vi "AMB_Monitor.vi"(0 "ObjHandle in":u32, 1 "CAN ID in":u32 format="%.0x", 2 "error in":errorcluster {"code" format="%.0x"}) -> (3 "ObjHandle out":u32, 4 "Data Array out":u8[](array[numeric]) format="%.0x", 5 "Data Length out":u8, 6 "error out":errorcluster {"code" format="%.0x"})   [LabVIEW 2017]
doc: "ALMA M&C Bus Read Monitor\nGets a monitor value on the specified CAN ID\nFirst clears the read queue of any stale messages\ntransmits the monitor requests and waits up to 2ms\nfor a response. Timeout is signalled in error cluster."
panel:
  # "AMB Monitor and Control Bus\nGet Monitor Data"
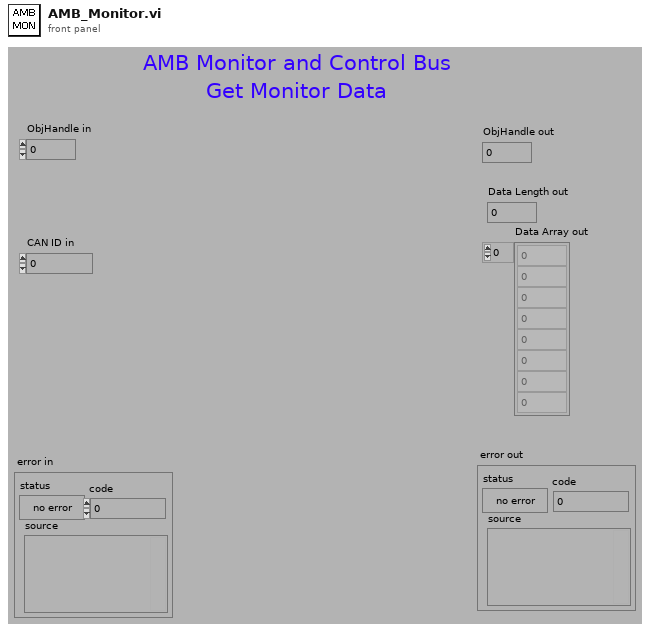
[diagram p1: front panel]
types:
  T1 = typedef "xobjhandle.ctl" = u32
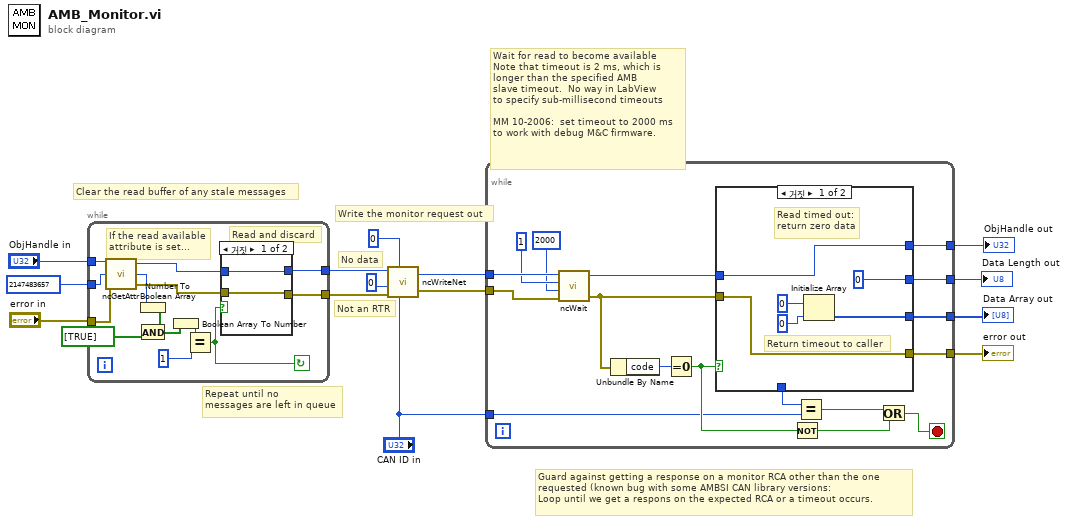
[diagram p0: block diagram]
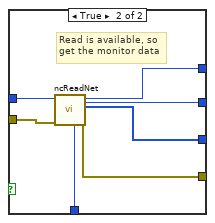
[diagram p2: hidden frame]
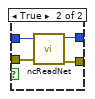
[diagram p3: hidden frame]
diagram:
  # "Guard against getting a response on a monitor RCA other than the one \nrequested (known bug with some AMBSI CAN library versions:\nLoop until we get a respons on the expected RCA or a timeout occurs."
  # "Wait for read to become available\nNote that timeout is 2 ms, which is\nlonger than the specified AMB\nslave timeout.  No way in LabView\nto specify sub-millisecond timeouts\n\nMM 10-2006:  set timeout to 2000 ms\nto work with debug M&C firmware."
  # "Not an RTR"
  # "No data"
  # "Write the monitor request out"
  # "Repeat until no\nmessages are left in queue"
  # "Clear the read buffer of any stale messages"
  n1 = while {
    tunnel: u32 2147483657 -> [w15]
    tunnel: [w22] -> w3
    tunnel: [w23] -> w4
    tunnel: "error in" -> [w27]
    tunnel: "ObjHandle in" -> [w28]
    stop <- w21 continue-if-true
    # "Read and discard"
    # "If the read available\nattribute is set..."
    n2 = call <vilib>:"ncGetAttr.vi"("Error in"=w27, "AttrId"=w15, "ObjHandle in"=w28) -> ("Error out"=w24:errorcluster, "AttrValue"=w20:u32, "ObjHandle out"=w25:T1)
    n3 = Number To Boolean Array(number=w20) -> (Boolean array=w19:bool[])
    n4 = And(x=w19, y=bool[] [TRUE]) -> (x .and. y?=w17:bool[])
    n5 = Boolean Array To Number(Boolean array=w17) -> (number=w16:u32)
    n6 = Equal?(x=w16, y=u32 1) -> (x = y?=w21:bool)
    n7 = case shown="거짓" w21 {
      tunnel: w25 -> [w30 w34]
      tunnel: w24 -> [w29 w33]
      tunnel: [w30 w32] -> w23
      tunnel: [w29 w31] -> w22
      frame False {
      }
      frame True {
        n8 = call <vilib>:"ncReadNet.vi"("ObjHandle in"=w34, "Error in"=w33) -> ("ObjHandle out"=w32:T1, "Error out"=w31:errorcluster)  [unwired: 2 in, 5 out]
      }
    }
  }
  n9 = call <vilib>:"ncWriteNet.vi"("ArbitrationId"="CAN ID in", "DataLength"=u32 0, "Error in"=w3, "IsRemote"=u8 0, "ObjHandle in"=w4) -> ("Error out"=w11:errorcluster, "ObjHandle out"=w12:T1)  [unwired: 1 in]
  n10 = while {
    tunnel: w12 -> [w51]
    tunnel: w11 -> [w48]
    tunnel: [w46] -> w10
    tunnel: [w45] -> w9
    tunnel: [w44] -> w8
    tunnel: [w43] -> w7
    tunnel: "CAN ID in" -> [w35]
    stop <- w39 stop-if-true
    n11 = call <vilib>:"ncWait.vi"("Error in"=w48, "Timeout"=2000, "DesiredState"=u32 1, "ObjHandle in"=w51) -> ("Error out"=w42:errorcluster, "ObjHandle out"=w47:T1)  [unwired: 1 out]
    n12 = Unbundle By Name(w42) -> ("code"=w41:i32)
    n13 = Equal To 0?(x=w41) -> (x = 0?=w36:bool)
    n14 = case shown="거짓" w36 {
      tunnel: w47 -> [w57 w64]
      tunnel: w42 -> [w56 w63]
      tunnel: [w56 w62] -> w43
      tunnel: [w57 w61] -> w44
      tunnel: [w52 w60] -> w46
      tunnel: [0 w59] -> w45
      tunnel: [_ w58] -> w40
      frame False {
        # "Return timeout to caller"
        # "Read timed out:\nreturn zero data"
        n15 = Initialize Array(u8 0 ("Element Data"), 0 ("Dimension Size")) -> (w52:u8[])
      }
      frame True {
        # "Read is available, so\nget the monitor data"
        n16 = call <vilib>:"ncReadNet.vi"("ObjHandle in"=w64, "Error in"=w63) -> ("DataLength"=w59:u32, "ArbitrationId"=w58:u32, "ObjHandle out"=w61:T1, "Data"=w60:u8[], "Error out"=w62:errorcluster)  [unwired: 2 in, 2 out]
      }
    }
    n17 = Not(x=w36) -> (.not. x?=w37:bool)
    n18 = Equal?(x=w40, y=w35) -> (x = y?=w38:bool)
    n19 = Or(x=w38, y=w37) -> (x .or. y?=w39:bool)
  }
  "ObjHandle out" <- w8
  "error out" <- w7
  "Data Array out" <- w10
  "Data Length out" <- w9
